vi "Get BLISS_Delete Random from Array.vi"(11 "filepath array in":path[](array[path])) -> (1 "random deleted filepath":path, 3 "remaining array":path[](array[path]))   [LabVIEW 2020]
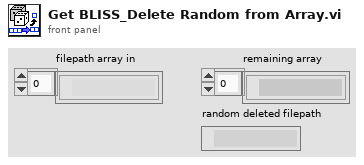
[diagram p1: front panel]
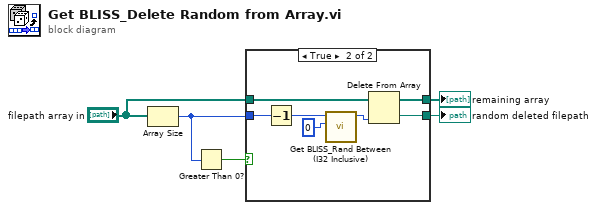
[diagram p0: block diagram]
diagram:
  n1 = Array Size(array="filepath array in") -> (size(s)=w5:i32)
  n2 = Greater Than 0?(x=w5) -> (x > 0?=w4:bool)
  n3 = case shown="True" w4 {
    tunnel: [w6 w10] -> w2
    tunnel: [_ w9] -> w1
    tunnel: "filepath array in" -> [w6 w7]
    tunnel: w5 -> [_ w8]
    frame False {
    }
    frame True {
      n4 = Decrement(x=w8) -> (x-1=w11:i32)
      n5 = call "Get BLISS_Rand Between (I32 Inclusive).vi"("lo limit (I32 inclusive)"=0 ("lower bound (0)"), "hi limit (I32 inclusive)"=w11) -> ("Result"=w13:i32)  [unwired: 9 in]
      n6 = Delete From Array(array=w7, index=w13) -> (deleted portion=w9:path, array with subset deleted=w10:path[])  [unwired: 1 in]
    }
  }
  "remaining array" <- w2
  "random deleted filepath" <- w1
